vi "Show_Save_Load_ XY_Data.vi"(2 "1D Array X":dbl[](array[numeric]) format="%.6f", 3 "1D Array Y":dbl[](array[numeric]) format="%.6f", 5 "error in":errorcluster, 6 "No. of digits X":i32=3 min=0, 7 "No. of digits Y":i16=2 min=0, 9 "Autoscale":bool, 11 "Names":string[](array[string])) -> (19 "error out":errorcluster)   [LabVIEW 2015]
doc: "This VI displays XY data in an XY Graph. If 1D Array X is an empty array, N X values are calculated with N = Size of 1D Array Y and Delta X = 1. No. of digits determines the resolution of Table and XY Graph. Data can be saved or loaded and a screen copy can be saved as JPG.\n\nIf data (1D Array X, 1D Array Y) are sent to the VI via the corresponding connectors, the VI will display the corresponding graphics after being called. To load data at runtime, press the Load data button. A dialog will pop up where a data file to open can be selected. The VI can read data in GCSArray, GCSTable and simple ASCII column format. Autoscale can be switched on or off. If Autoscale is off, the Y axis of the graph is scaled from 0-10. \n\nPress Save data to save data (file header and numerical data). Data will be saved in GCS Array format. The file header will contain information given in X axis name, Y axis name and Remarks. With Save panel a screen copy of this VI can be saved as a JPG file. XY Graph will show the Y values over the corresponding X values. Table contains the numerical values for X and Y. Press Exit to stop execution of this VI.\n\nValid for Analog systems, C-866, C-867, C-880, E-712, E-725, E-753, E-755, E-761, E-861, F-206, M-8X0. To support analog interfacing, VI must be present for E-816 also."
uses:
  <vilib>/Analysis/3filter.llb/Butterworth Filter (DBL).vi
  <vilib>/Analysis/NI_AALBase.lvlib
panel:
  in  "Filter options":T1={"Filter type"=enum."Lowpass", "Order"=5, "Sampling f"=1000.0, "High cutoff f"=0.45000000000000007, "Low cutoff f"=40.0} {"Low cutoff f" format="%0.4f"; "High cutoff f" format="%0.2f"; "Sampling f" format="%0.2f"}
  in  "Filter":bool
  out "File path":path=path "no path"
  out "error":bool
  in  "Save jpg":bool
  in  "Remarks":string
  in  "Y axis name":string
  in  "X axis name":string
  in  "Redraw":bool
  in  "Next frame":i32
  in  "Exit":bool
  in  "Save data":bool
  in  "Load data":bool
  out "Table":string[][](table)
  out "XY Graph":cluster{"1D Array X":dbl[], "1D Array Y":dbl[]}(graph)
  # "This vi displays XY data in a XY Graph. If \"1D Array X\" is an empty array, N X values are calculated with N = Size of \"1D Array Y\" and Delta X = 1. \nNo. of digits determines resolution of Table and XY Graph. Data can be saved or loaded and screen copy can be saved as JPG."
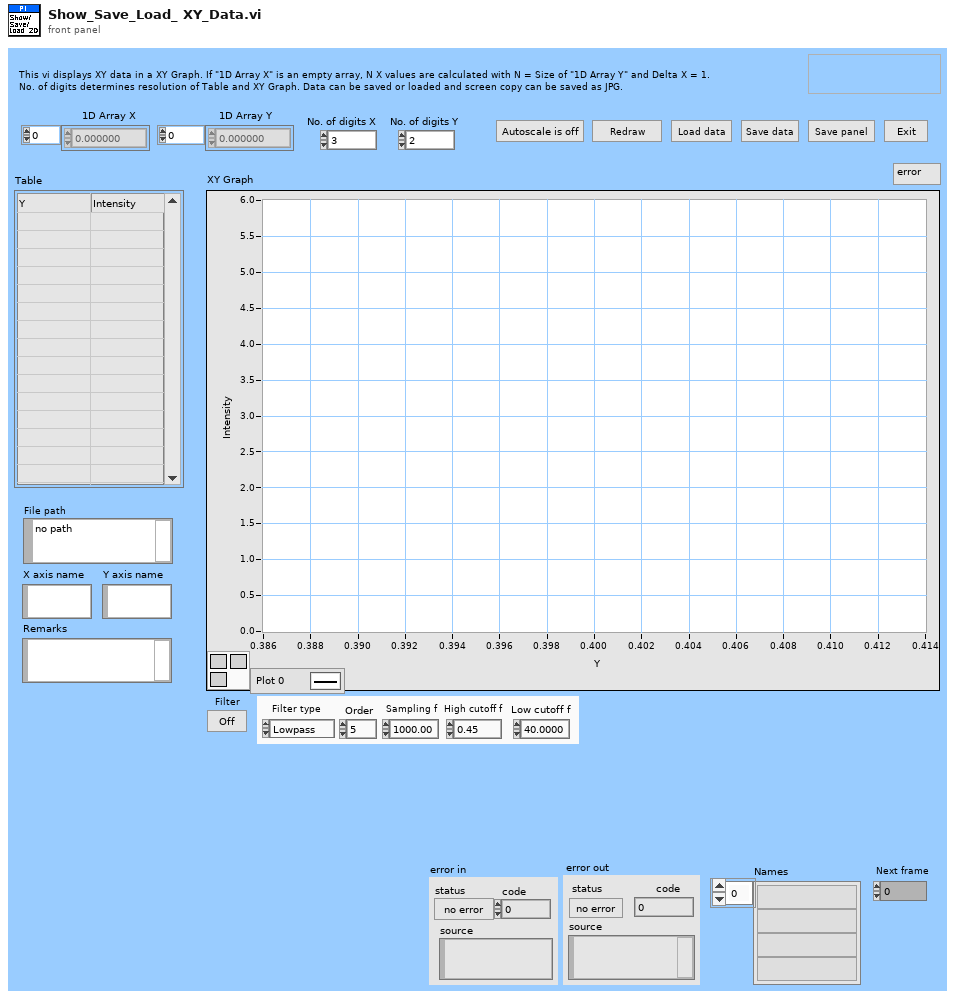
[diagram p1: front panel]
types:
  T1 = cluster{"Filter type":enum32{"Lowpass", "Highpass", "Bandpass", "Bandstop"}, "Order":i32, "Sampling f":dbl, "High cutoff f":dbl, "Low cutoff f":dbl}
  T2 = cluster{"Read/Write":bool, "Path":path, "Datastream":string, "ArrayName":string}
  T3 = cluster{"XName":string, "YName":string, "ZName":string}
  T4 = cluster{"Separator":string, "Remarks":string, "NDim":i32}
  T5 = cluster{"Read (F)/ Write":bool, "Path":path, "Datastream":string, "ArrayName":string}
  T6 = cluster{"Filter type":bool, "Order":bool, "Sampling f":bool, "High cutoff f":bool, "Low cutoff f":bool}
  T7 = typedef "LVRectTypeDef.ctl" = cluster{"Left":i16, "Top":i16, "Right":i16, "Bottom":i16}
  T8 = enum32{"Lowpass", "Highpass", "Bandpass", "Bandstop"}
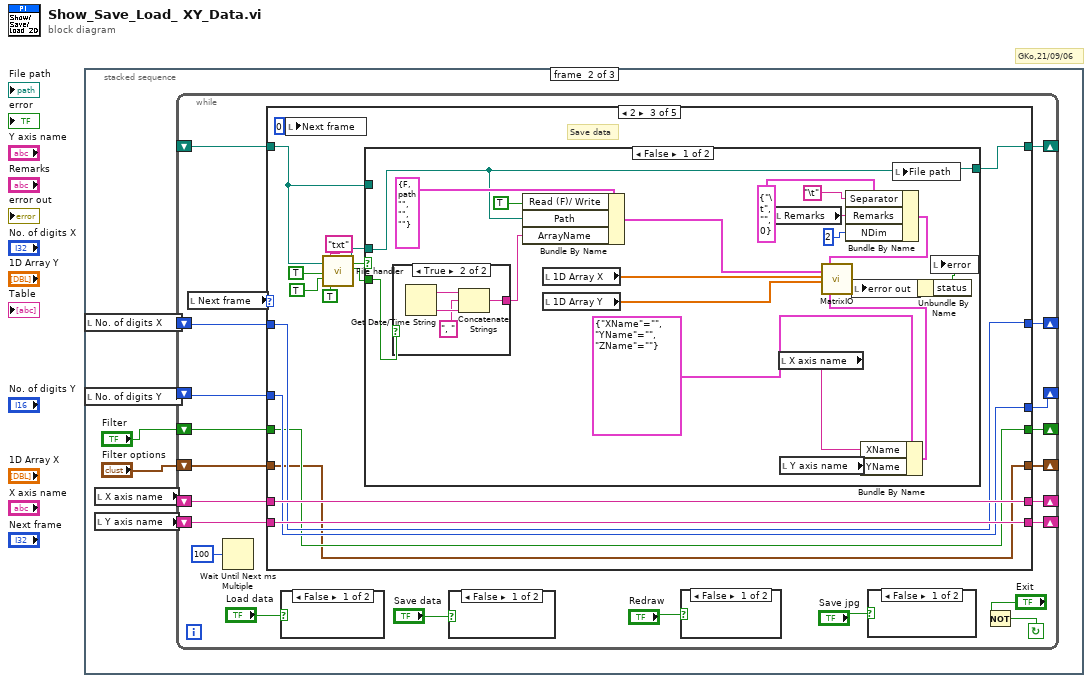
[diagram p0: block diagram]
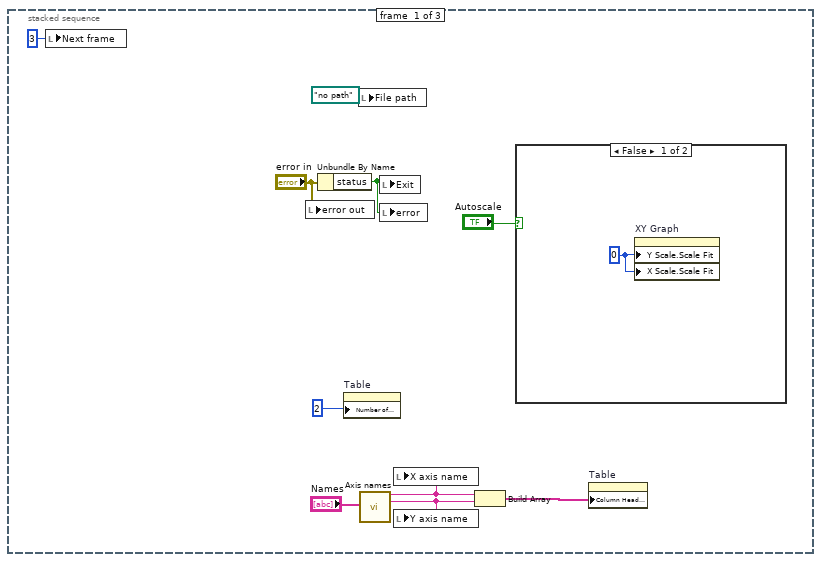
[diagram p2: hidden frame]
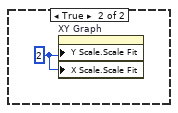
[diagram p3: hidden frame]
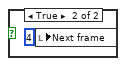
[diagram p4: hidden frame]
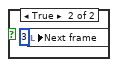
[diagram p5: hidden frame]
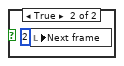
[diagram p6: hidden frame]
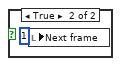
[diagram p7: hidden frame]
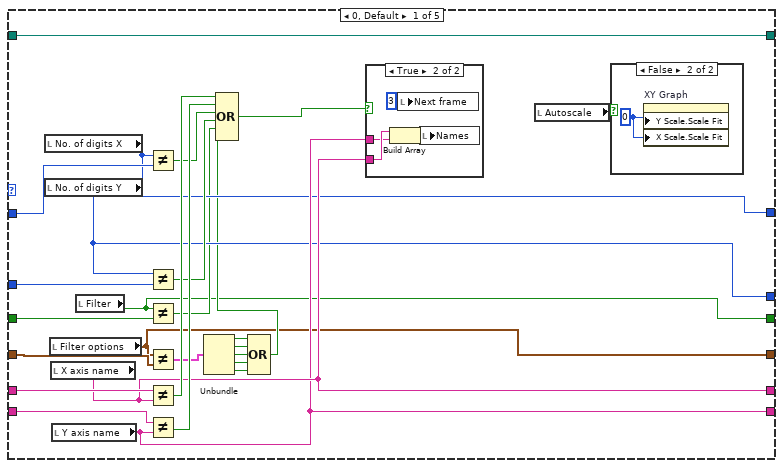
[diagram p8: hidden frame]
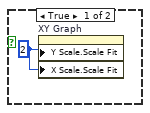
[diagram p10: hidden frame]
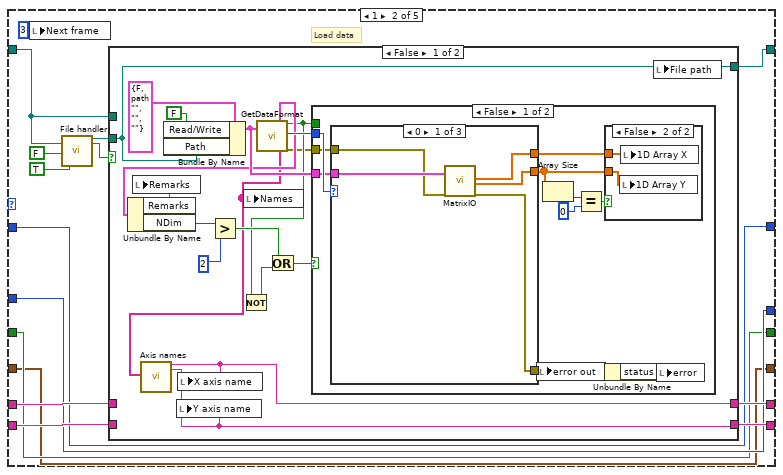
[diagram p11: hidden frame]
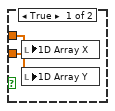
[diagram p12: hidden frame]
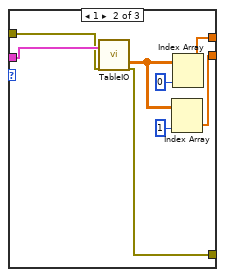
[diagram p13: hidden frame]
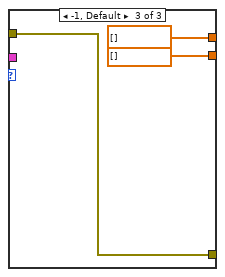
[diagram p14: hidden frame]
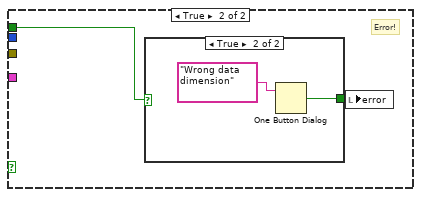
[diagram p15: hidden frame]
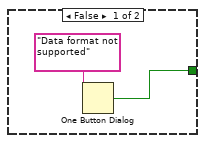
[diagram p16: hidden frame]
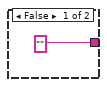
[diagram p18: hidden frame]
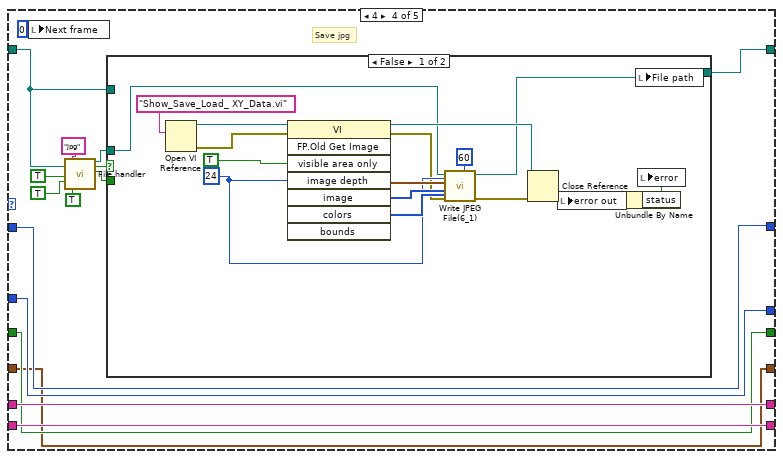
[diagram p20: hidden frame]
diagram:
  # "GKo,21/09/06"
  n1 = stacked-sequence {
    frame #0 {
      n2 = local write "Next frame"(3 ("Next frame")) -> ()
      n3 = local write "error out"("error in") -> ()
      n4 = Unbundle By Name("error in") -> ("status"=w3:bool)
      n5 = property on="Table" class="Tbl (strict)"("Number of Columns"=u32 2 ("Write Attribute")) -> ()  [unwired: 2 in, 2 out]
      n6 = local write "File path"(path "no path" ("File path")) -> ()
      n7 = call "Axis names.vi"("Names"="Names") -> ("X axis name"=w5:string, "Y axis name"=w4:string)  [unwired: 16 in, 1 out]
      n8 = local write "Exit"(w3) -> ()
      n9 = local write "error"(w3) -> ()
      n10 = local write "X axis name"(w5) -> ()
      n11 = local write "Y axis name"(w4) -> ()
      n12 = Build Array(w5, w4) -> (w7:string[])
      n13 = case shown="False" "Autoscale" {
        frame False {
          w11 = u8 0 ("Write Attribute")
          n14 = property on="XY Graph" class="XYGraph (strict)"("Y Scale.Scale Fit"=w11, "X Scale.Scale Fit"=w11) -> ()  [unwired: 2 in, 2 out]
        }
        frame True {
          w12 = u8 2 ("Write Attribute")
          n15 = property on="XY Graph" class="XYGraph (strict)"("Y Scale.Scale Fit"=w12, "X Scale.Scale Fit"=w12) -> ()  [unwired: 2 in, 2 out]
        }
      }
      n16 = property on="Table" class="Tbl (strict)"("Column Header Strings[]"=w7) -> ()  [unwired: 2 in, 2 out]
    }
    frame #1 {
      n17 = local read "No. of digits X"() -> (w16:i32)
      n18 = local read "No. of digits Y"() -> (w15:i16)
      n19 = local read "X axis name"() -> (w18:string)
      n20 = local read "Y axis name"() -> (w17:string)
      n21 = while {
        shift-left: w15 -> [w26]
        shift-right: [w23] -> _
        shift-left: w16 -> [w25]
        shift-right: [w24] -> _
        shift-left: w17 -> [w29]
        shift-right: [w27] -> _
        shift-left: w18 -> [w30]
        shift-right: [w28] -> _
        shift-left: _ -> [w32]
        shift-right: [w33] -> _
        shift-right: [w19] -> _
        shift-left: "Filter" -> [w22]
        shift-right: [w20] -> _
        shift-left: "Filter options" -> [w21]
        stop <- w39 continue-if-true
        n22 = local read "Next frame"() -> (w38:i32)
        n23 = Wait Until Next ms Multiple(millisecond multiple=u32 100) -> ()  [unwired: 1 out]
        n24 = case shown="2" w38 {
          tunnel: [w70 w81 w152 w199 w230] -> w33
          tunnel: w32 -> [w70 w80 w151 w192 w230]
          tunnel: w30 -> [w67 w86 w158 w196 _]
          tunnel: w29 -> [w66 w85 w157 w195 _]
          tunnel: [w64 w88 w158 w196 w229] -> w28
          tunnel: [w63 w87 w157 w195 w228] -> w27
          tunnel: w26 -> [w58 w83 w155 w193 _]
          tunnel: w25 -> [w60 w84 w156 w194 _]
          tunnel: [w59 w84 w156 w194 w226] -> w24
          tunnel: [w57 w83 w155 w193 w227] -> w23
          tunnel: w22 -> [w55 w79 w150 w191 w223]
          tunnel: w21 -> [w54 w78 w149 w190 w224]
          tunnel: [w46 w78 w149 w190 w224] -> w20
          tunnel: [w45 w79 w150 w191 w223] -> w19
          frame 0, Default {
            n25 = local read "No. of digits X"() -> (w59:i32)
            n26 = local read "No. of digits Y"() -> (w57:i16)
            n27 = local read "Filter options"() -> (w46:T1)
            n28 = local read "X axis name"() -> (w64:string)
            n29 = local read "Y axis name"() -> (w63:string)
            n30 = local read "Filter"() -> (w45:bool)
            n31 = Not Equal?(x=w59, y=w60) -> (x != y?=w62:bool)
            n32 = Not Equal?(x=w57, y=w58) -> (x != y?=w61:bool)
            n33 = Not Equal?(x=w45, y=w55) -> (x != y?=w56:bool)
            n34 = Not Equal?(x=w46, y=w54) -> (x != y?=w53:T6)
            n35 = Not Equal?(x=w67, y=w64) -> (x != y?=w69:bool)
            n36 = Not Equal?(x=w66, y=w63) -> (x != y?=w68:bool)
            n37 = Unbundle(w53) -> ("Filter type"=w52:bool, "Order"=w51:bool, "Sampling f"=w50:bool, "High cutoff f"=w49:bool, "Low cutoff f"=w48:bool)
            n38 = Compound Arithmetic op=OR(w52, w51, w50, w49, w48) -> (w47:bool)
            n39 = Compound Arithmetic op=OR(w69, w68, w62, w61, w56, w47) -> (w65:bool)
            n40 = case shown="True" w65 {
              tunnel: w64 -> [_ w75]
              tunnel: w63 -> [_ w74]
              frame False {
              }
              frame True {
                n41 = Build Array(w75, w74) -> (w73:string[])
                n42 = local write "Next frame"(3 ("Next frame")) -> ()
                n43 = local write "Names"(w73) -> ()
              }
            }
            n44 = local read "Autoscale"() -> (w71:bool)
            n45 = case shown="False" w71 {
              frame True {
                w76 = u8 2 ("Write Attribute")
                n46 = property on="XY Graph" class="XYGraph (strict)"("Y Scale.Scale Fit"=w76, "X Scale.Scale Fit"=w76) -> ()  [unwired: 2 in, 2 out]
              }
              frame False {
                w77 = u8 0 ("Write Attribute")
                n47 = property on="XY Graph" class="XYGraph (strict)"("Y Scale.Scale Fit"=w77, "X Scale.Scale Fit"=w77) -> ()  [unwired: 2 in, 2 out]
              }
            }
          }
          frame 1 {
            # "Load data"
            n48 = local write "Next frame"(3 ("Next frame")) -> ()
            n49 = call "File handler.vi"("Path in"=w80, "Read (F) or write (T)?"=FALSE, "With dialog?"=TRUE ("With dialog")) -> ("Path out"=w82:path, "Cancelled?"=w90:bool)  [unwired: 14 in, 1 out]
            n50 = case shown="False" w90 {
              tunnel: w82 -> [w93 _]
              tunnel: [w96 w148] -> w88
              tunnel: [w95 w147] -> w87
              tunnel: w86 -> [_ w148]
              tunnel: w85 -> [_ w147]
              tunnel: [w93 w146] -> w81
              tunnel: w80 -> [_ w146]
              frame False {
                n51 = Bundle By Name(cluster=T2 {"Read/Write"=FALSE, "Path"=path "", "Datastream"="", "ArrayName"=""} ("IOSource"), "Read/Write"=FALSE ("Bundle Element"), "Path"=w93) -> (w107:T2)
                n52 = call "GetDataFormat.vi"("IOSource"=w107) -> ("Header out"=w104:T4, "Names out"=w97:string[], "DataOK"=w101:bool, "Data Type"=w108:i32, "error out"=w94:errorcluster)  [unwired: 11 in, 3 out]
                n53 = Unbundle By Name(w104) -> ("Remarks"=w99:string, "NDim"=w105:i32)
                n54 = local write "Remarks"(w99) -> ()
                n55 = call "Axis names.vi"("Names"=w97) -> ("X axis name"=w96:string, "Y axis name"=w95:string)  [unwired: 16 in, 1 out]
                n56 = local write "Y axis name"(w95) -> ()
                n57 = local write "X axis name"(w96) -> ()
                n58 = Greater?(x=w105, y=2) -> (0:w103:bool)
                n59 = Not(x=w101) -> (.not. x?=w102:bool)
                n60 = local write "Names"(w97) -> ()
                n61 = Or(x=w103, y=w102) -> (x .or. y?=w100:bool)
                n62 = case shown="False" w100 {
                  tunnel: w108 -> [w119 _]
                  tunnel: w107 -> [w118 _]
                  tunnel: w101 -> [_ w141]
                  tunnel: w94 -> [w112 _]
                  frame False {
                    n63 = case shown="0" w119 {
                      tunnel: w118 -> [w128 w136 _]
                      tunnel: [w127 w132 dbl[] [] ("XArray out")] -> w114
                      tunnel: [w126 w131 dbl[] [] ("YArray out")] -> w113
                      tunnel: w112 -> [w125 w130 w137]
                      tunnel: [w124 w129 w137] -> w111
                      frame 0 {
                        n64 = call "MatrixIO.vi"("IOSource"=w128, "error in"=w125) -> ("XArray out"=w127:dbl[], "YArray out"=w126:dbl[], "error out"=w124:errorcluster)  [unwired: 11 in, 4 out]
                      }
                      frame 1 {
                        n65 = call "TableIO.vi"("IOSource"=w136, "error in"=w130) -> ("Table out"=w134:dbl[][], "error out"=w129:errorcluster)  [unwired: 12 in, 4 out]
                        n66 = Index Array(array=w134, index (col)=1 ("Index")) -> (element=w131:dbl[])  [unwired: 1 in]
                        n67 = Index Array(array=w134, index (col)=0 ("Index")) -> (element=w132:dbl[])  [unwired: 1 in]
                      }
                      frame -1, Default {
                      }
                    }
                    n68 = local write "error out"(w111) -> ()
                    n69 = Array Size(array=w113) -> (size(s)=w117:i32)
                    n70 = Equal?(x=w117, y=0) -> (x = y?=w115:bool)
                    n71 = case shown="False" w115 {
                      tunnel: w114 -> [w121 w122]
                      tunnel: w113 -> [w120 w123]
                      frame True {
                        n72 = local write "1D Array X"(w120) -> ()
                        n73 = local write "1D Array Y"(w121) -> ()
                      }
                      frame False {
                        n74 = local write "1D Array Y"(w123) -> ()
                        n75 = local write "1D Array X"(w122) -> ()
                      }
                    }
                    n76 = Unbundle By Name(w111) -> ("status"=w110:bool)
                    n77 = local write "error"(w110) -> ()
                  }
                  frame True {
                    # "Error!"
                    n78 = case shown="True" w141 {
                      tunnel: [w142 w144] -> w140
                      frame False {
                        n79 = One Button Dialog(message="Data format not supported") -> (true=w142:bool)  [unwired: 1 in]
                      }
                      frame True {
                        n80 = One Button Dialog(message="Wrong data dimension") -> (true=w144:bool)  [unwired: 1 in]
                      }
                    }
                    n81 = local write "error"(w140) -> ()
                  }
                }
                n82 = local write "File path"(w93) -> ()
              }
              frame True {
              }
            }
          }
          frame 2 {
            # "Save data"
            n83 = local write "Next frame"(0 ("Next frame")) -> ()
            n84 = call "File handler.vi"("Path in"=w151, "Read (F) or write (T)?"=TRUE ("New File?"), "Write new File?"=TRUE, "Extension"="txt", "With dialog?"=TRUE ("With dialog")) -> ("Path out"=w153:path, "Cancelled?"=w163:bool, "Data added?"=w160:bool)  [unwired: 12 in]
            n85 = case shown="False" w163 {
              tunnel: w153 -> [w166 _]
              tunnel: w160 -> [w170 _]
              tunnel: [w166 w189] -> w152
              tunnel: w151 -> [_ w189]
              frame False {
                n86 = case shown="True" w170 {
                  tunnel: ["" ("ArrayName") w185] -> w169
                  frame False {
                  }
                  frame True {
                    n87 = Get Date/Time String() -> (date string=w188:string, time string=w187:string)  [unwired: 3 in]
                    n88 = Concatenate Strings(w188, ", " ("Substring"), w187) -> (w185:string)
                  }
                }
                n89 = Bundle By Name(cluster=T5 {"Read (F)/ Write"=FALSE, "Path"=path "", "Datastream"="", "ArrayName"=""} ("IOSource"), "Read (F)/ Write"=TRUE, "Path"=w166, "ArrayName"=w169) -> (w179:T5)
                n90 = local read "1D Array X"() -> (w182:dbl[])
                n91 = local read "1D Array Y"() -> (w183:dbl[])
                n92 = local read "Remarks"() -> (w177:string)
                n93 = local read "X axis name"() -> (w173:string)
                n94 = local read "Y axis name"() -> (w172:string)
                n95 = Bundle By Name(cluster=T4 {"Separator"="\t", "Remarks"="", "NDim"=0} ("Header in"), "Separator"="\t", "Remarks"=w177, "NDim"=2) -> (w175:T4)
                n96 = Bundle By Name(cluster=T3 {"XName"="", "YName"="", "ZName"=""} ("Data names"), "XName"=w173, "YName"=w172) -> (w171:T3)
                n97 = call "MatrixIO.vi"("IOSource"=w179, "XArray in"=w182, "YArray in"=w183, "Header in"=w175, "Data names"=w171) -> ("error out"=w168:errorcluster)  [unwired: 8 in, 6 out]
                n98 = local write "error out"(w168) -> ()
                n99 = local write "File path"(w166) -> ()
                n100 = Unbundle By Name(w168) -> ("status"=w167:bool)
                n101 = local write "error"(w167) -> ()
              }
              frame True {
              }
            }
          }
          frame 4 {
            # "Save jpg"
            n102 = local write "Next frame"(0 ("Next frame")) -> ()
            n103 = call "File handler.vi"("Path in"=w192, "Read (F) or write (T)?"=TRUE ("New File?"), "Write new File?"=TRUE, "Extension"="jpg", "With dialog?"=TRUE ("With dialog")) -> ("Path out"=w198:path, "Cancelled?"=w204:bool, "Data added?"=w201:bool)  [unwired: 12 in]
            n104 = case shown="False" w204 {
              tunnel: w198 -> [w209 _]
              tunnel: w201 -> [_ _]
              tunnel: [w206 w222] -> w199
              tunnel: w192 -> [_ w222]
              frame False {
                w213 = 24 ("image depth")
                n105 = Open VI Reference(vi path="Show_Save_Load_ XY_Data.vi") -> (vi reference=w219:refnum<vi>, error out=w220:errorcluster)  [unwired: 5 in]
                n106 = invoke class="VI" method="FP.Old Get Image"(reference=w219, error in=w220, "visible area only"=TRUE, "image depth"=w213) -> (reference out=w221:refnum<vi>, error out=w212:errorcluster, "image"=w216:u8[], "colors"=w218:u32[], "bounds"=w217:T7)  [unwired: 4 in, 3 out]
                n107 = call <vilib>:"Write JPEG File(6_1).vi"("quality (80)"=60, "color table"=w218, "depth"=w213, "error in (no error)"=w212, "flattened image data"=w216, "rect"=w217, "path to JPEG file"=w209) -> ("error out"=w211:errorcluster, "path"=w206:path)  [unwired: 3 in]
                n108 = Close Reference(reference=w221, error in (no error)=w211) -> (error out=w208:errorcluster)
                n109 = local write "error out"(w208) -> ()
                n110 = Unbundle By Name(w208) -> ("status"=w207:bool)
                n111 = local write "File path"(w206) -> ()
                n112 = local write "error"(w207) -> ()
              }
              frame True {
              }
            }
          }
          frame 3 {
            w241 = FALSE ("use system decimal point (T)")
            # "Redraw"
            n113 = local read "1D Array Y"() -> (w238:dbl[])
            n114 = local read "1D Array X"() -> (w233:dbl[])
            n115 = local read "X axis name"() -> (w229:string)
            n116 = local read "Y axis name"() -> (w228:string)
            n117 = local write "Next frame"(0 ("Next frame")) -> ()
            n118 = Array Size(array=w233) -> (size(s)=w236:i32)
            n119 = Equal?(x=w236, y=0) -> (x = y?=w234:bool)
            n120 = case shown="False" w234 {
              tunnel: [w253 w271] -> w225
              tunnel: [w252 w270] -> w226
              tunnel: [w251 w268] -> w240
              tunnel: w238 -> [w248 w267]
              tunnel: w233 -> [w251 _]
              tunnel: w223 -> [w249 w265]
              tunnel: w224 -> [w247 w264]
              frame False {
                n121 = case shown="True" w249 {
                  tunnel: w248 -> [w254 w255]
                  tunnel: [w254 w262] -> w250
                  tunnel: w247 -> [_ w256]
                  frame False {
                  }
                  frame True {
                    n122 = Unbundle By Name(w256) -> ("Filter type"=w261:T8, "Order"=w260:i32, "Sampling f"=w259:dbl, "High cutoff f"=w258:dbl, "Low cutoff f"=w257:dbl)
                    n123 = call-poly <vilib>:"Butterworth Filter.vi"("init/cont (init:F)"=TRUE, "order"=w260, "filter type"=w261, "low cutoff freq: fl"=w257, "high cutoff freq: fh"=w258, "sampling freq: fs"=w259, "X"=w255) -> ("Filtered X"=w262:dbl[])  [unwired: 1 in, 1 out]
                  }
                }
                n124 = Bundle("1D Array X"=w251, "Filtered X"=w250) -> (w253:cluster{"1D Array X":dbl[], "Filtered X":dbl[]})  [unwired: 1 in]
                n125 = local read "No. of digits X"() -> (w252:i32)
              }
              frame True {
                w270 = 0
                n126 = Array Size(array=w267) -> (size(s)=w273:i32)
                n127 = Initialize Array(0 ("Element Data"), w273) -> (w274:i32[])
                n128 = local write "No. of digits X"(w270) -> ()
                n129 = for {
                  N: w273 -> [_]
                  shift-right: [w285] -> w269
                  shift-left: w274 -> [w287]
                  i -> [w286]
                  n130 = Replace Array Subset(array=w287, new element=w286, index=w286) -> (w285:i32[])
                }
                n131 = To Double Precision Float(number=w269) -> (double precision float=w268:dbl[])
                n132 = case shown="True" w265 {
                  tunnel: w267 -> [w275 w284]
                  tunnel: [w275 w282] -> w266
                  tunnel: w264 -> [_ w276]
                  frame False {
                  }
                  frame True {
                    n133 = Unbundle By Name(w276) -> ("Filter type"=w281:T8, "Order"=w280:i32, "Sampling f"=w279:dbl, "High cutoff f"=w278:dbl, "Low cutoff f"=w277:dbl)
                    n134 = call-poly <vilib>:"Butterworth Filter.vi"("init/cont (init:F)"=TRUE, "order"=w280, "filter type"=w281, "low cutoff freq: fl"=w277, "high cutoff freq: fh"=w278, "sampling freq: fs"=w279, "X"=w284) -> ("Filtered X"=w282:dbl[])  [unwired: 1 in, 1 out]
                  }
                }
                n135 = local write "1D Array X"(w268) -> ()
                n136 = Bundle(w268, "Filtered X"=w266) -> (w271:cluster{dbl[], "Filtered X":dbl[]})  [unwired: 1 in]
              }
            }
            "XY Graph" <- w225
            n137 = Build Array(w229, w228) -> (w231:string[])
            n138 = property on="Table" class="Tbl (strict)"("Column Header Strings[]"=w231) -> ()  [unwired: 2 in, 2 out]
            n139 = local read "No. of digits Y"() -> (w227:i16)
            n140 = Number To Fractional String(use system decimal point (T)=w241, number=w240, precision (6)=w226) -> (F-format string=w244:string[])  [unwired: 1 in]
            n141 = Number To Fractional String(use system decimal point (T)=w241, number=w238, precision (6)=w227) -> (F-format string=w243:string[])  [unwired: 1 in]
            n142 = Build Array(w244, w243) -> (w242:string[][])
            n143 = Transpose 2D Array(2D array=w242) -> (transposed array=w237:string[][])
            n144 = local read "Autoscale"() -> (w232:bool)
            n145 = local write "Table"(w237) -> ()
            n146 = case shown="True" w232 {
              frame True {
                w245 = u8 2 ("Write Attribute")
                n147 = property on="XY Graph" class="XYGraph (strict)"("Y Scale.Scale Fit"=w245, "X Scale.Scale Fit"=w245) -> ()  [unwired: 2 in, 2 out]
              }
              frame False {
                w246 = u8 0 ("Write Attribute")
                n148 = property on="XY Graph" class="XYGraph (strict)"("Y Scale.Scale Fit"=w246, "X Scale.Scale Fit"=w246) -> ()  [unwired: 2 in, 2 out]
              }
            }
            n149 = property on="XY Graph" class="XYGraph (strict)"("X Scale.Display Format:Precision"=w226, "X Scale.Name Label.Text"=w229, "Y Scale.Name Label.Text"=w228) -> ()  [unwired: 2 in, 2 out]
          }
        }
        n150 = case shown="False" "Load data" {
          frame False {
          }
          frame True {
            n151 = local write "Next frame"(1) -> ()
          }
        }
        n152 = case shown="False" "Save data" {
          frame False {
          }
          frame True {
            n153 = local write "Next frame"(2) -> ()
          }
        }
        n154 = case shown="False" "Redraw" {
          frame False {
          }
          frame True {
            n155 = local write "Next frame"(3 ("Next frame")) -> ()
          }
        }
        n156 = case shown="False" "Save jpg" {
          frame False {
          }
          frame True {
            n157 = local write "Next frame"(4 ("Next frame")) -> ()
          }
        }
        n158 = Not(x="Exit") -> (.not. x?=w39:bool)
      }
    }
    frame #2 {
      n159 = local write "Exit"(FALSE ("stop")) -> ()
    }
  }
